vi "Read Configuration and Measurements.vi"(8 "error in (no error)":errorcluster, 11 "HFP Gen in":refnum<class "PL HFP Generator.lvclass">) -> (0 "error out":errorcluster, 1 "measurements":T1 {"rf power"."Ppump, W" items=["500", "1000", "2000", "3000", "4000", "6000", "8000"]; "SWR timer state" items=["off"=0, "counting"=2, "counting and skipping"=3, "protection"=4]; "power ramp state" items=["off", "ramp up", "full power", "ramp down", "off, awaiting reset"]}, 2 "configuration":T2 {"modulation mode" items=["off"=0, "internal full"=2, "internal partial"=3, "external full"=4, "external partial"=5]; "power ramp mode" items=["off", "ramp up", "ramp up and down", "ramp down"]; "control mode" items=["Pload", "Pfwd"]}, 3 "HFP Gen out":refnum<class "PL HFP Generator.lvclass">)   [LabVIEW 2015, in "PL HFP Generator.lvclass"]
doc: "Reads device configuration and measurements."
uses:
  PL HFP Generator.lvclass
  <vilib>/plasmapper/PL Modbus Client/PL Modbus Client.lvclass
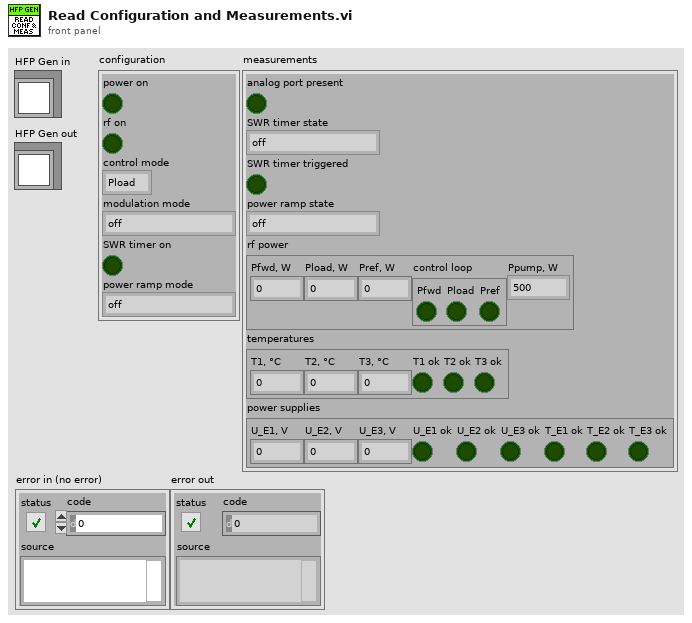
[diagram p1: front panel]
types:
  T1 = cluster{"analog port present":bool, "SWR timer state":u8, "SWR timer triggered":bool, "power ramp state":u8, "rf power":cluster{"Pfwd, W":dbl, "Pload, W":dbl, "Pref, W":dbl, "control loop":cluster{"Pfwd":bool, "Pload":bool, "Pref":bool}, "Ppump, W":u8}, "temperatures":cluster{"T1, °C":dbl, "T2, °C":dbl, "T3, °C":dbl, "T1 ok":bool, "T2 ok":bool, "T3 ok":bool}, "power supplies":cluster{"U_E1, V":dbl, "U_E2, V":dbl, "U_E3, V":dbl, "U_E1 ok":bool, "U_E2 ok":bool, "U_E3 ok":bool, "T_E1 ok":bool, "T_E2 ok":bool, "T_E3 ok":bool}}
  T2 = cluster{"power on":bool, "rf on":bool, "control mode":u8, "modulation mode":u8, "SWR timer on":bool, "power ramp mode":u8}
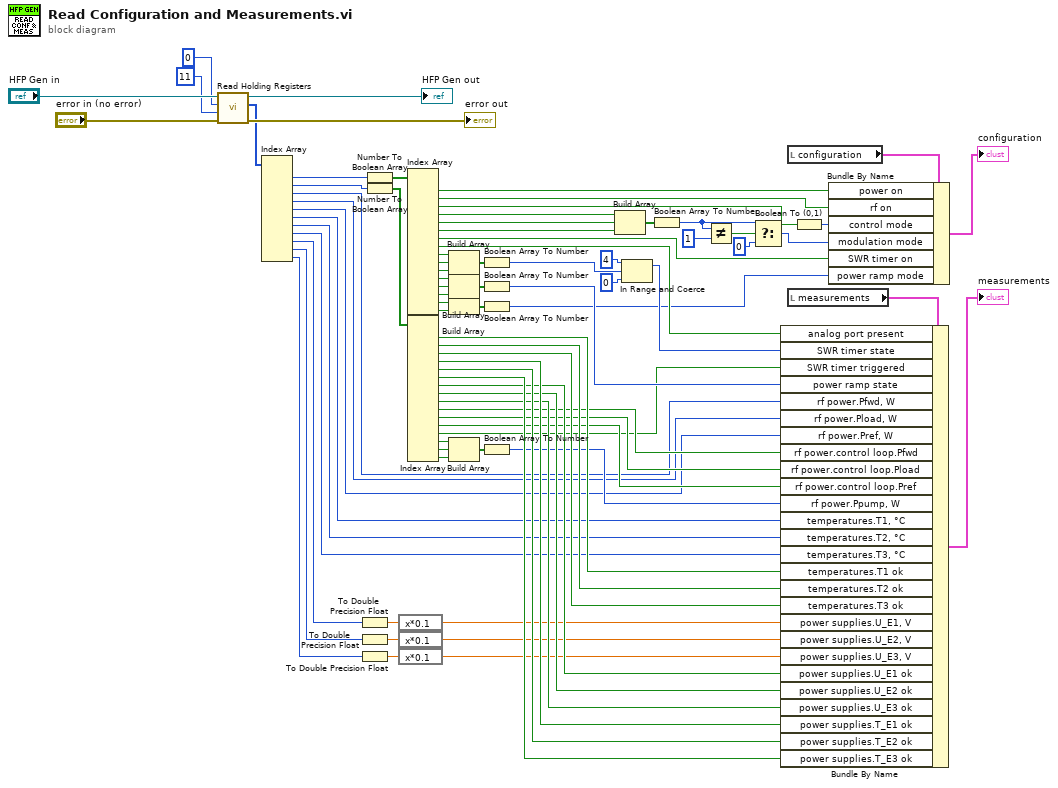
[diagram p0: block diagram]
diagram:
  n1 = call <vilib>:"Read Holding Registers.vi"("error in (no error)"="error in (no error)", "number of holding registers"=u16 11, "address"=u16 0, "MODBUS in"="HFP Gen in") -> ("error out"=→"error out":errorcluster, "values"=w70:u16[], "MODBUS out"=→"HFP Gen out":refnum<class "PL HFP Generator.lvclass">)  [unwired: 5 in]
  n2 = Index Array(array=w70) -> (element #1=w69:u16, element #2=w68:u16, element #3=w15:u16, element #4=w14:u16, element #5=w13:u16, element #6=w12:u16, element #7=w11:u16, element #8=w10:u16, element #9=w8:u16, element #10=w2:u16, element #11=w1:u16)  [unwired: 11 in]
  n3 = To Double Precision Float(number=w8) -> (double precision float=w9:dbl)
  n4 = To Double Precision Float(number=w2) -> (double precision float=w7:dbl)
  n5 = To Double Precision Float(number=w1) -> (double precision float=w6:dbl)
  n6 = Number To Boolean Array(number=w69) -> (Boolean array=w67:bool[])
  n7 = Number To Boolean Array(number=w68) -> (Boolean array=w34:bool[])
  n8 = expression code="x*0.1"(w9) -> (w5:dbl)
  n9 = expression code="x*0.1"(w7) -> (w4:dbl)
  n10 = expression code="x*0.1"(w6) -> (w3:dbl)
  n11 = Index Array(array=w67) -> (element #1=w66:bool, element #2=w65:bool, element #3=w64:bool, element #4=w62:bool, element #5=w60:bool, element #6=w61:bool, element #7=w59:bool, element #8=w52:bool, element #9=w51:bool, element #10=w50:bool, element #11=w49:bool, element #12=w43:bool, element #13=w42:bool, element #14=w41:bool, element #15=w40:bool, element #16=w39:bool)  [unwired: 16 in]
  n12 = Index Array(array=w34) -> (element #1=w33:bool, element #2=w32:bool, element #3=w31:bool, element #4=w30:bool, element #5=w29:bool, element #6=w28:bool, element #7=w27:bool, element #8=w26:bool, element #9=w25:bool, element #10=w24:bool, element #11=w23:bool, element #12=w22:bool, element #13=w21:bool, element #14=w20:bool, element #15=w19:bool, element #16=w18:bool)  [unwired: 16 in]
  n13 = Build Array(w51, w50, w49) -> (w48:bool[])
  n14 = Build Array(w43, w42, w41) -> (w38:bool[])
  n15 = Build Array(w40, w39) -> (w37:bool[])
  n16 = Build Array(w20, w19, w18) -> (w17:bool[])
  n17 = Boolean Array To Number(Boolean array=w48) -> (number=w47:u32)
  n18 = Boolean Array To Number(Boolean array=w38) -> (number=w36:u32)
  n19 = Boolean Array To Number(Boolean array=w37) -> (number=w35:u32)
  n20 = Boolean Array To Number(Boolean array=w17) -> (number=w16:u32)
  n21 = Build Array(w62, w60, w61) -> (w58:bool[])
  n22 = In Range and Coerce(upper limit=u32 4, x=w47, lower limit=u32 0) -> (coerced(x)=w44:u32)  [unwired: 1 out]
  n23 = Boolean Array To Number(Boolean array=w58) -> (number=w55:u32)
  n24 = Not Equal?(x=w55, y=u32 1) -> (x != y?=w56:bool)
  n25 = Select(t=w55, s=w56, f=u32 0) -> (s? t:f=w53:u32)
  n26 = local read "configuration"() -> (w72:T2)
  n27 = local read "measurements"() -> (w74:T1)
  n28 = Bundle By Name(cluster=w74, "analog port present"=w52, "SWR timer state"=w44, "SWR timer triggered"=w21, "power ramp state"=w36, "rf power.Pfwd, W"=w15, "rf power.Pload, W"=w14, "rf power.Pref, W"=w13, "rf power.control loop.Pfwd"=w24, "rf power.control loop.Pload"=w23, "rf power.control loop.Pref"=w22, "rf power.Ppump, W"=w16, "temperatures.T1, °C"=w12, "temperatures.T2, °C"=w11, "temperatures.T3, °C"=w10, "temperatures.T1 ok"=w33, "temperatures.T2 ok"=w32, "temperatures.T3 ok"=w31, "power supplies.U_E1, V"=w5, "power supplies.U_E2, V"=w4, "power supplies.U_E3, V"=w3, "power supplies.U_E1 ok"=w27, "power supplies.U_E2 ok"=w26, "power supplies.U_E3 ok"=w25, "power supplies.T_E1 ok"=w30, "power supplies.T_E2 ok"=w29, "power supplies.T_E3 ok"=w28) -> (→"measurements":T1)
  n29 = Boolean To (0,1)(Boolean=w64) -> (0, 1=w63:i16)
  n30 = Bundle By Name(cluster=w72, "power on"=w66, "rf on"=w65, "control mode"=w63, "modulation mode"=w53, "SWR timer on"=w59, "power ramp mode"=w35) -> (→"configuration":T2)
